vi "NF WF1973_74 CHAN Mode.vi"(6 "Read(F)":bool, 8 "error in (no error)":errorcluster caption="Error IN", 10 "Channel Mode(Independent)":i32(ring) items=["Independent", "Phase", "Tone", "Ratio", "Differential"], 11 "VISAsession":refnum<visa-resource-name>) -> (0 "error out":errorcluster caption="Error OUT", 2 "Query Mode":string, 3 "CopyVISAsession":refnum<visa-resource-name>)   [LabVIEW 2010]
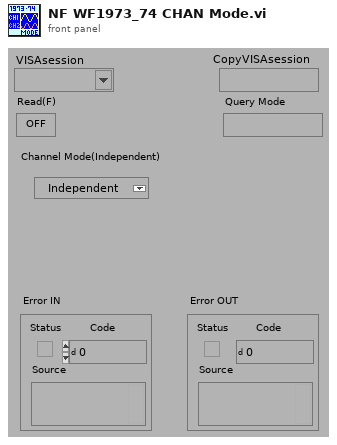
[diagram p1: front panel]
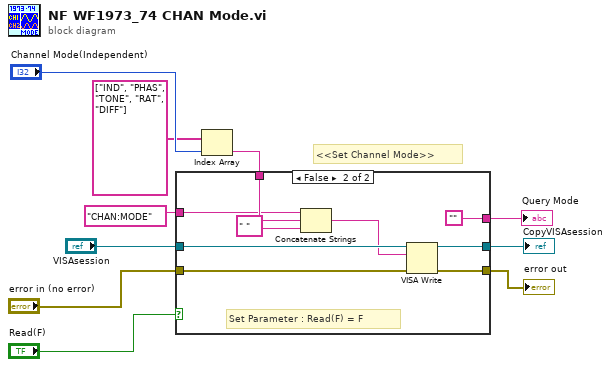
[diagram p0: block diagram]
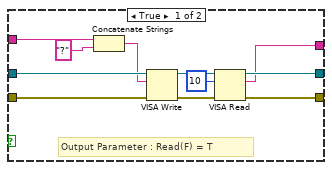
[diagram p2: hidden frame]
diagram:
  # "<<Set Channel Mode>>"
  n1 = Index Array(array=string[] ["IND", "PHAS", "TONE", "RAT", "DIFF"], index="Channel Mode(Independent)") -> (element=w1:string)
  n2 = case shown="FALSE" "Read(F)" {
    tunnel: "VISAsession" -> [w21 w30]
    tunnel: [w18 w27] -> w9
    tunnel: [w17 w28] -> w8
    tunnel: "error in (no error)" -> [w16 w29]
    tunnel: "CHAN:MODE" ("文字列") -> [w14 w22]
    tunnel: [w11 ""] -> w4
    tunnel: w1 -> [_ w24]
    frame True {
      # "Output Parameter : Read(F) = T"
      n3 = Concatenate Strings(w14, "?" ("形式文字列")) -> (w12:string)
      n4 = VISA Write(VISA resource name=w21, write buffer=w12, error in (no error)=w16) -> (VISA resource name out=w19:refnum<visa-resource-name>, error out=w20:errorcluster)  [unwired: 1 out]
      n5 = VISA Read(VISA resource name=w19, byte count=u32 10 ("バイトカウント（0）"), error in (no error)=w20) -> (VISA resource name out=w18:refnum<visa-resource-name>, read buffer=w11:string, error out=w17:errorcluster)  [unwired: 1 out]
    }
    frame False {
      # "Set Parameter : Read(F) = F"
      n6 = Concatenate Strings(w22, " ", w24) -> (w25:string)
      n7 = VISA Write(VISA resource name=w30, write buffer=w25, error in (no error)=w29) -> (VISA resource name out=w27:refnum<visa-resource-name>, error out=w28:errorcluster)  [unwired: 1 out]
    }
  }
  "error out" <- w8
  "CopyVISAsession" <- w9
  "Query Mode" <- w4
